vi "Deserialize CD XML FIle.vi"(8 "Error In":errorcluster caption="error in", 11 "XML Path":path) -> (0 "Error Out":errorcluster caption="error in", 3 "Custom Device .NET Ref Out":refnum<k24>)   [LabVIEW 2019, in "VeriStand Custom Device XML Parser.lvlib"]
doc: "Deserializes the provided custom device XML file and returns a reference to the file in memory."
uses:
  VeriStand Custom Device XML Parser.lvlib
  NationalInstruments.VeriStand.XMLReader
  <vilib>/Utility/sysdir.llb/System Directory Type.ctl
  subVI/Global Settings.vi
  Configuration Tool.lvlib
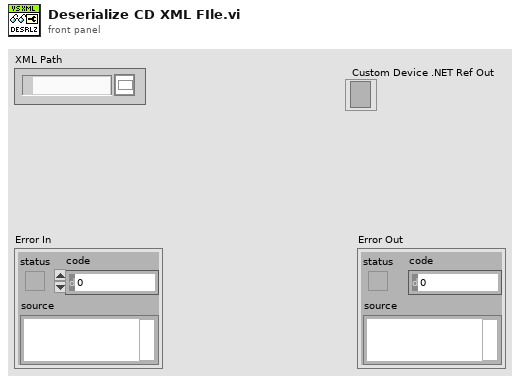
[diagram p1: front panel]
types:
  T1 = typedef "System Directory Type.ctl" = i32
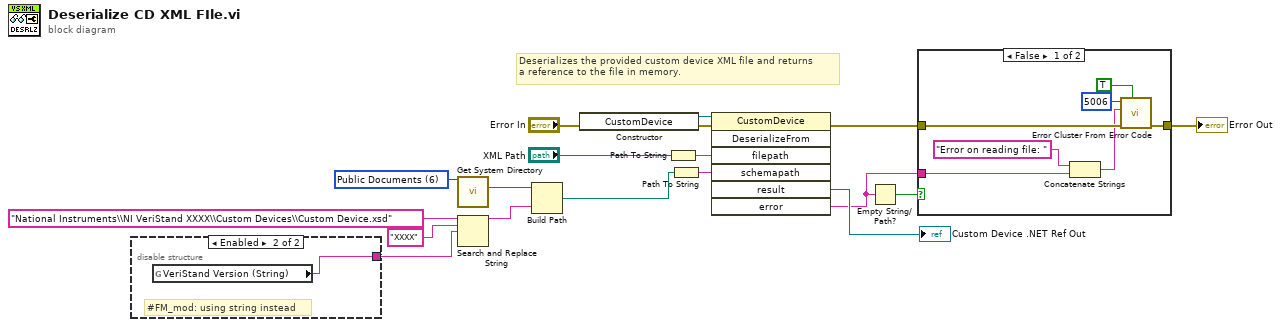
[diagram p0: block diagram]
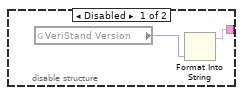
[diagram p2: hidden frame]
diagram:
  w14 = T1 6 items=["User Home"=0, "User Desktop"=1, "User Documents"=2, "User Application Data"=3, "User Preferences"=4, "User Temporary"=5, "Public Documents"=6, "Public Application Data"=7, "Public Preferences"=8, "Public Cache"=13, "System Core Libraries"=9, "System Installed Libraries"=10, "Application Files"=11, "Boot Volume Root"=12] ("system directory type")
  # "Deserializes the provided custom device XML file and returns\na reference to the file in memory."
  n1 = disable-structure shown="Enabled" {
    disable-tunnel: [w19 w21] -> w1
    frame Disabled {
      n2 = global read "Global Settings.vi" "VeriStand Version"() -> (w20:enum16{"2013", "2014", "2015", "2016"})
      n3 = Format Into String(w20) -> (resulting string=w19:string)  [unwired: 3 in, 1 out]
    }
    frame Enabled {
      # "#FM_mod: using string instead"
      n4 = global read "Global Settings.vi" "VeriStand Version (String)"() -> (w21:string)
    }
  }
  n5 = call <vilib>:"Get System Directory.vi"("system directory type"=w14) -> ("system directory"=w13:path)  [unwired: 10 in]
  n6 = Search and Replace String(input string="National Instruments\\NI VeriStand XXXX\\Custom Devices\\Custom Device.xsd", search string="XXXX", replace string=w1) -> (result string=w8:string)  [unwired: 5 in, 3 out]
  n7 = Build Path(base path=w13, name or relative path=w8) -> (appended path=w12:path)
  n8 = constructor class="CustomDevice"(error in="Error In") -> (reference out=w16:refnum<k24>, error out=w6:errorcluster)  [unwired: 2 in, 1 out]
  n9 = Path To String(path="XML Path") -> (string=w15:string)
  n10 = Path To String(path=w12) -> (string=w11:string)
  n11 = invoke class="CustomDevice" method="DeserializeFrom"(reference=w16, error in=w6, "filepath"=w15, "schemapath"=w11) -> (error out=w3:errorcluster, "result"=→"Custom Device .NET Ref Out":refnum<k24>, "error"=w4:string)  [unwired: 3 in, 4 out]
  n12 = Empty String/Path?(string/path=w4) -> (empty?=w5:bool)
  n13 = case shown="False" w5 {
    tunnel: w4 -> [w27 _]
    tunnel: w3 -> [w26 w29]
    tunnel: [w23 w29] -> w2
    frame False {
      n14 = Concatenate Strings("Error on reading file: " ("string"), w27) -> (w24:string)
      n15 = call <vilib>:"Error Cluster From Error Code.vi"("show call chain? (False)"=TRUE, "error in (no error)"=w26, "error message (\"\")"=w24, "error code (0)"=5006) -> ("error out"=w23:errorcluster)  [unwired: 5 in]
    }
    frame True {
    }
  }
  "Error Out" <- w2
